vi "Enqueue Depth2Read.vi"(8 "Error In":errorcluster, 10 "Depth":u16, 11 "Name":string) -> (0 "Error Out":errorcluster, 2 "Data":variant)   [LabVIEW 2019, in "SR_2000.lvlib"]
uses:
  SR_2000.lvlib
  Queue/Queue.lvlib
  Data Error Notifier/Data and Error Notifier.lvlib
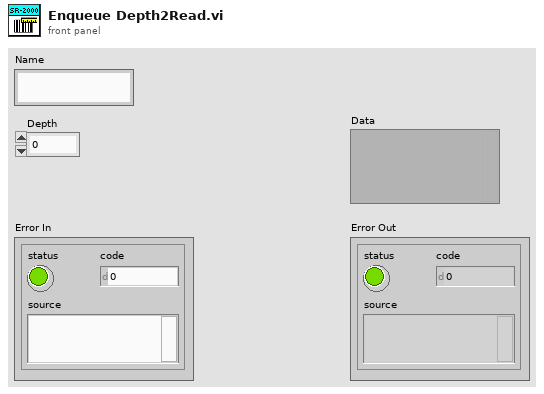
[diagram p1: front panel]
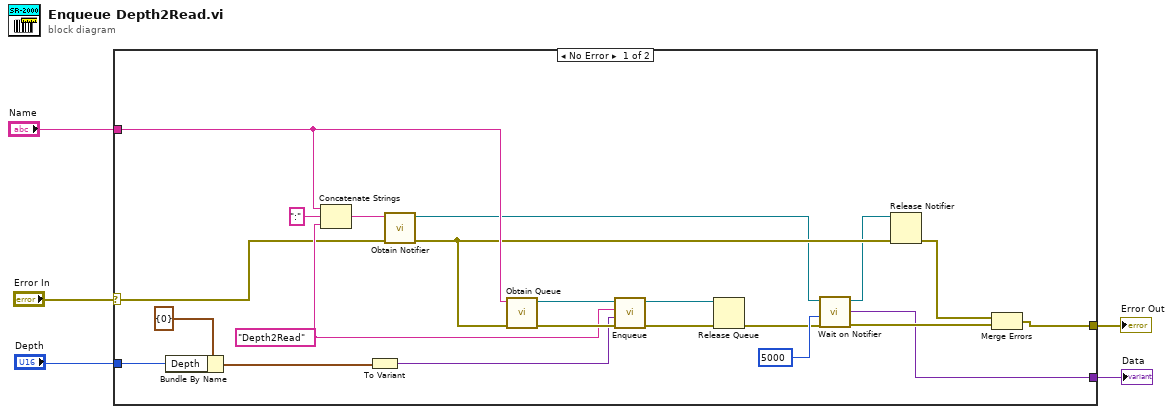
[diagram p0: block diagram]
diagram:
  n1 = case shown="No Error" "Error In" {
    selector: "Error In" -> [w16 w28]
    tunnel: [w19 w28] -> w4
    tunnel: "Name" -> [w26 _]
    tunnel: "Depth" -> [w8 _]
    tunnel: [w9 _] -> w1
    frame No Error {
      w24 = "Depth2Read" ("Message")
      n2 = Bundle By Name(cluster=cluster{"Depth":u16} {"Depth"=0}, "Depth"=w8) -> (w6:cluster{"Depth":u16})
      n3 = Concatenate Strings(w26, ":" ("string"), w24) -> (w17:string)
      n4 = To Variant(anything=w6) -> (Variant=w18:variant)
      n5 = call "Obtain Notifier.vi"("Error In"=w16, "Name"=w17) -> ("Error Out"=w15:errorcluster, "notifier out"=w14:refnum<notifier>)  [unwired: 8 in]
      n6 = call "Obtain Queue.vi"("Error In"=w15, "Name"=w26) -> ("Error Out"=w27:errorcluster, "queue out"=w22:refnum<queue>)  [unwired: 8 in]
      n7 = call "Enqueue.vi"("Error In"=w27, "Data"=w18, "Message"=w24, "queue in"=w22) -> ("Error Out"=w23:errorcluster, "queue out"=w21:refnum<queue>)  [unwired: 6 in]
      n8 = Release Queue(queue=w21, error in (no error)=w23) -> (error out=w12:errorcluster)  [unwired: 1 in, 2 out]
      n9 = call "Wait on Notifier.vi"("Error In"=w12, "timeout in ms (-1)"=5000, "notifier in"=w14) -> ("Error Out"=w10:errorcluster, "Data"=w9:variant, "notifier out"=w11:refnum<notifier>)  [unwired: 6 in]
      n10 = Release Notifier(notifier=w11, error in (no error)=w15) -> (error out=w20:errorcluster)  [unwired: 1 in, 2 out]
      n11 = Merge Errors(w20, w10) -> (w19:errorcluster)
    }
    frame Error {
    }
  }
  "Error Out" <- w4
  "Data" <- w1
